vi "event_structure.vi"() -> ()   [LabVIEW 2023]
panel:
  out "Array 2":bool[](array[boolean])
  in  "operation":enum16{"AND", "OR", "XOR"}(ring)
  out "Boolean 48":bool
  out "Boolean 47":bool
  out "Boolean 46":bool
  out "Boolean 45":bool
  out "Boolean 44":bool
  out "Boolean 43":bool
  out "Boolean 42":bool
  out "Boolean 41":bool
  in  "Boolean 40":bool
  in  "Boolean 39":bool
  in  "Boolean 38":bool
  in  "Boolean 37":bool
  in  "Boolean 36":bool
  in  "Boolean 35":bool
  in  "Boolean 34":bool
  in  "Boolean 33":bool
  in  "Boolean 32":bool
  in  "Boolean 31":bool
  in  "Boolean 30":bool
  in  "Boolean 29":bool
  in  "Boolean 28":bool
  in  "Boolean 27":bool
  in  "Boolean 26":bool
  in  "Boolean 25":bool
  in  "check":bool
  in  "stop":bool
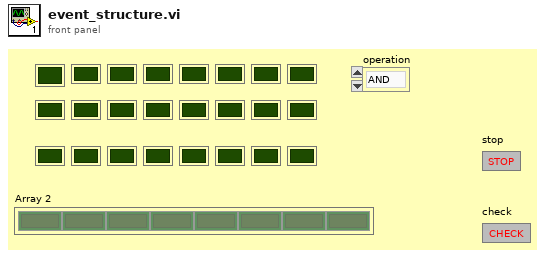
[diagram p1: front panel]
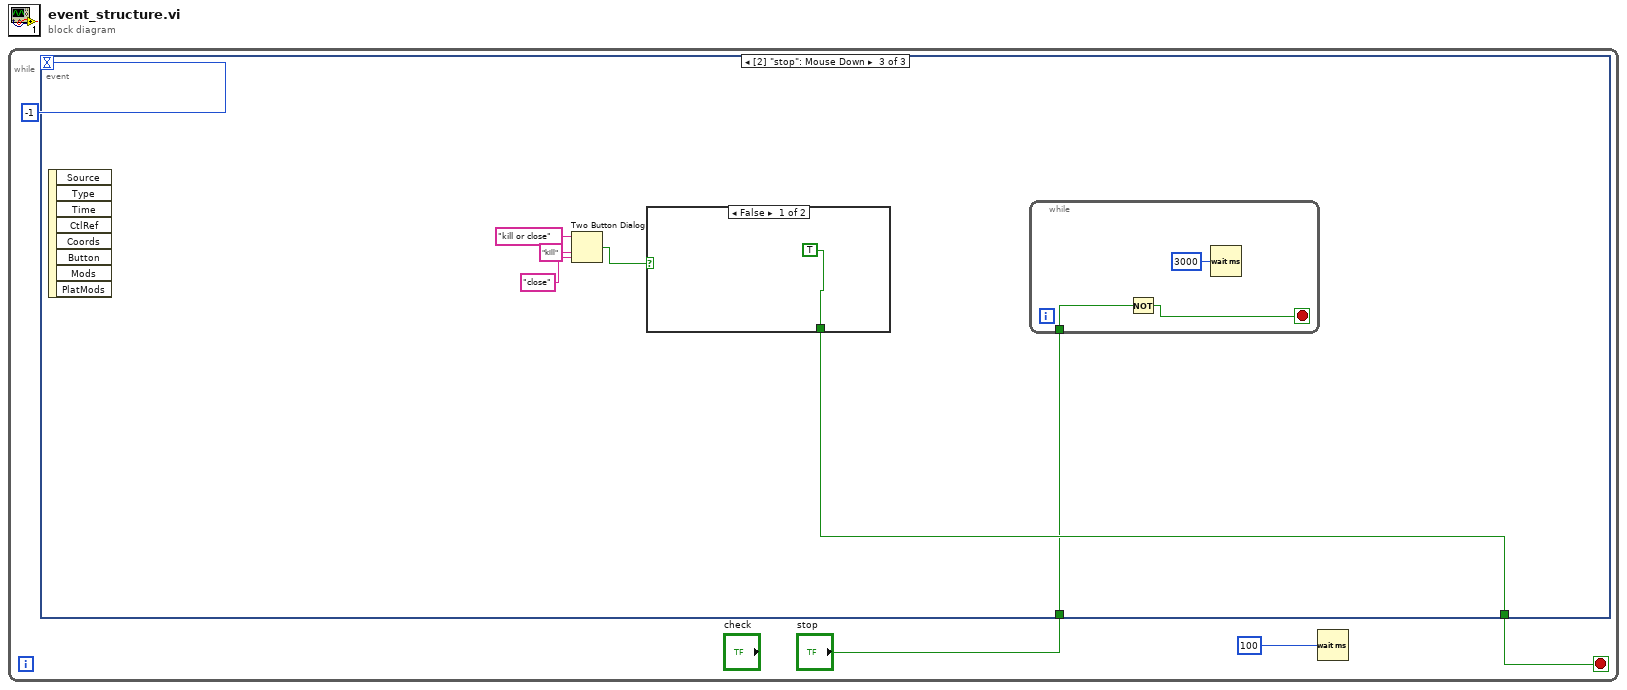
[diagram p0: block diagram]
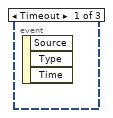
[diagram p2: hidden frame]
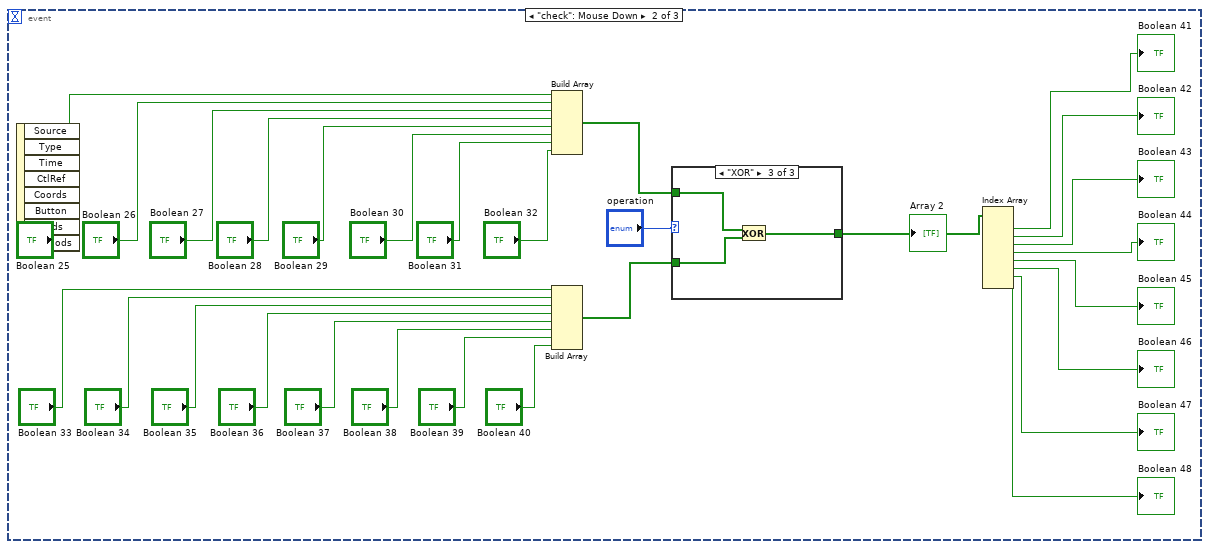
[diagram p3: hidden frame]
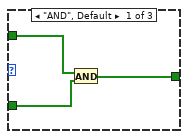
[diagram p4: hidden frame]
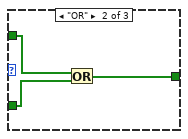
[diagram p5: hidden frame]
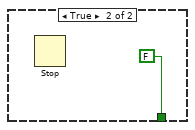
[diagram p6: hidden frame]
diagram:
  n1 = while {
    stop <- w2 stop-if-true
    n2 = event shown="[2] \"stop\": Mouse Down" {
      selector: _ -> [_ _ _]
      dyn-events: _ -> [_ _ _]
      timeout: -1 -> [_ _ _]
      tunnel: [_ _ w43] -> w2
      tunnel: "stop" -> [_ _ w42]
      event Timeout {
        n3 = event-data() -> ()  [unwired: 1 in, 3 out]
      }
      event "check": Mouse Down {
        n4 = event-data() -> ()  [unwired: 1 in, 8 out]
        n5 = Build Array("Boolean 25", "Boolean 26", "Boolean 27", "Boolean 28", "Boolean 29", "Boolean 30", "Boolean 31", "Boolean 32") -> (w14:bool[])
        n6 = Build Array("Boolean 33", "Boolean 34", "Boolean 35", "Boolean 36", "Boolean 37", "Boolean 38", "Boolean 39", "Boolean 40") -> (w15:bool[])
        n7 = case shown="\"XOR\"" "operation" {
          tunnel: w15 -> [w34 w38 w40]
          tunnel: w14 -> [w35 w37 w41]
          tunnel: [w33 w36 w39] -> w13
          frame "AND", Default {
            n8 = And(x=w35, y=w34) -> (x .and. y?=w33:bool[])
          }
          frame "OR" {
            n9 = Or(x=w37, y=w38) -> (x .or. y?=w36:bool[])
          }
          frame "XOR" {
            n10 = Exclusive Or(1:w40, 2:w41) -> (0:w39:bool[])
          }
        }
        "Array 2" <- w13
        n11 = Index Array(array=w13) -> (element #1=→"Boolean 41":bool, element #2=→"Boolean 42":bool, element #3=→"Boolean 43":bool, element #4=→"Boolean 44":bool, element #5=→"Boolean 45":bool, element #6=→"Boolean 46":bool, element #7=→"Boolean 47":bool, element #8=→"Boolean 48":bool)  [unwired: 8 in]
      }
      event "stop": Mouse Down {
        n12 = event-data() -> ()  [unwired: 1 in, 8 out]
        n13 = Two Button Dialog(message="kill or close", 1:"close" ("F button name (\"Cancel\")"), 2:"kill" ("T button name (\"OK\")")) -> (T button?=w44:bool)
        n14 = case shown="False" w44 {
          tunnel: [TRUE FALSE] -> w43
          frame False {
          }
          frame True {
            n15 = Stop() -> ()  [unwired: 1 in]
          }
        }
        n16 = while {
          tunnel: w42 -> [w49]
          stop <- w48 stop-if-true
          n17 = Not(x=w49) -> (.not. x?=w48:bool)
          n18 = Wait (ms)(milliseconds to wait=u32 3000) -> ()  [unwired: 1 out]
        }
      }
    }
    n19 = Wait (ms)(milliseconds to wait=100) -> ()  [unwired: 1 out]
  }
